vi "ReGenerate BFS Items.vi"(9 "Split Level":i32, 11 "Tree in":refnum<class "Tree.lvclass">) -> (0 "BFS Items Array":cluster{"Array of Single Level":T1[]}[](array[cluster]), 2 "Split Out":T1[](array[typedef]), 3 "Tree out":refnum<class "Tree.lvclass">)   [LabVIEW 2024, in "Tree.lvclass"]
uses:
  Tree.lvclass
  Type Def/Single Level.ctl
  Type Def/Tree Item.ctl
  Tree.lvclass/Tree.ctl
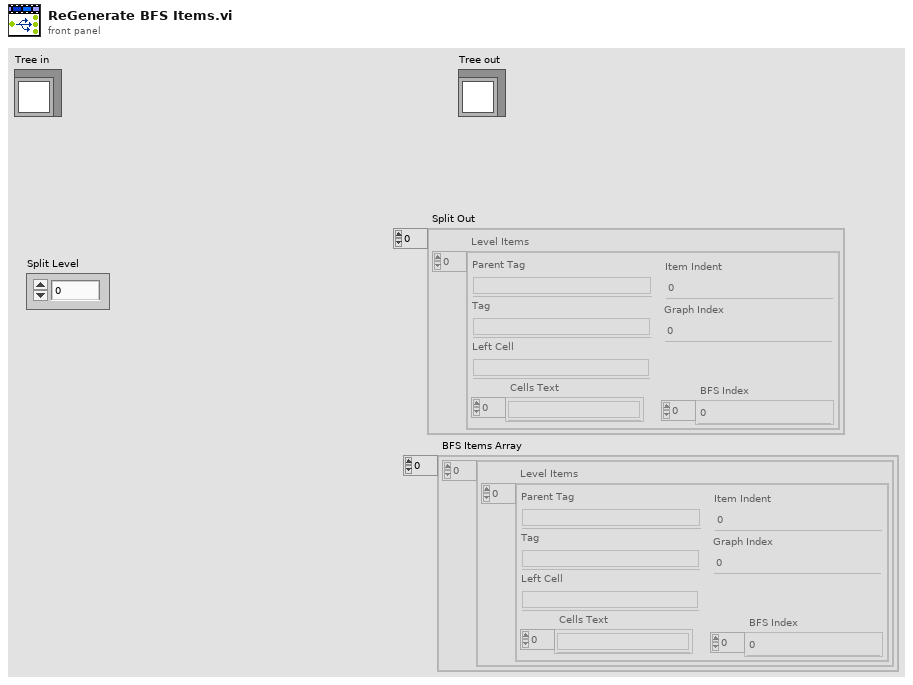
[diagram p1: front panel]
types:
  T1 = typedef "Single Level.ctl" = cluster{"Level Items":T2[]}
  T2 = typedef "Tree Item.ctl" = cluster{"Parent Tag":string, "Tag":string, "Left Cell":string, "Cells Text":string[], "BFS Index":i32[], "Graph Index":i32, "Item Indent":i32}
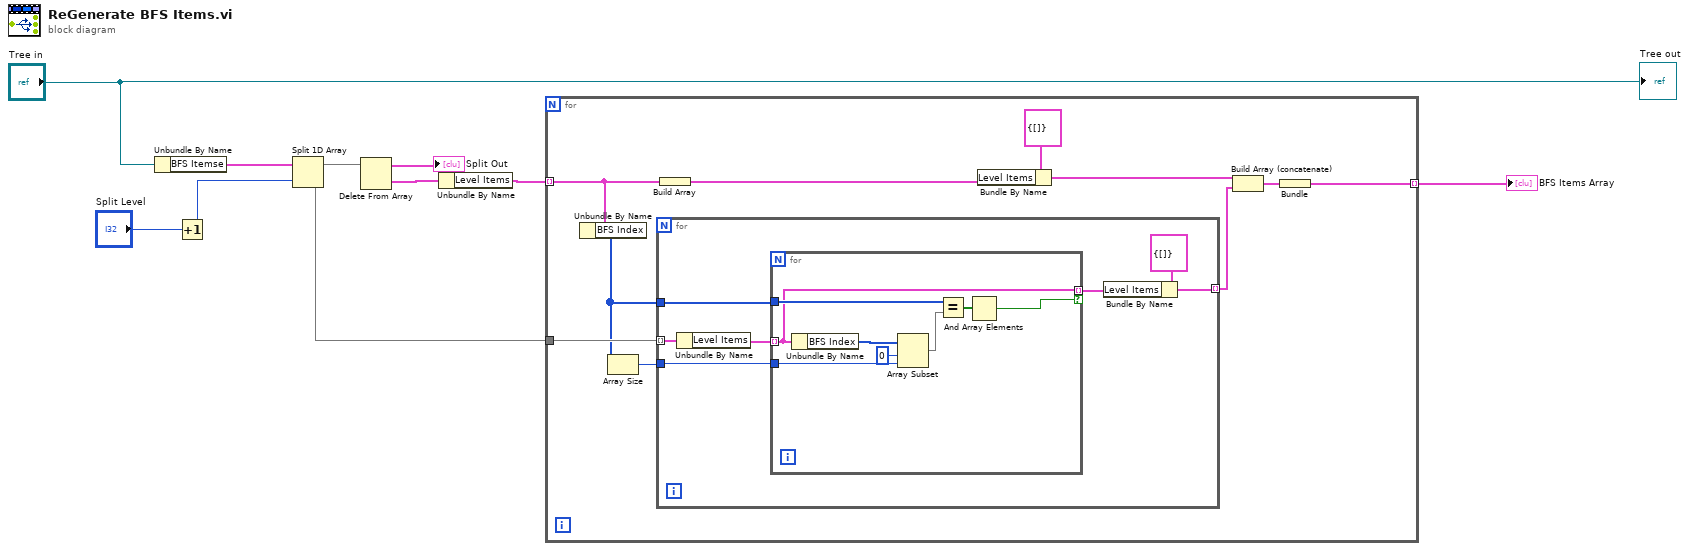
[diagram p0: block diagram]
diagram:
  n1 = Unbundle By Name("Tree in") -> ("BFS Itemse"=w8:T1[])
  n2 = Increment(x="Split Level") -> (x+1=w7:i32)
  n3 = Split 1D Array(array=w8, index=w7) -> (first subarray=w4:T1[], second subarray=w5:T1[])
  n4 = Delete From Array(array=w4) -> (deleted portion=w3:T1, array with subset deleted=→"Split Out":T1[])  [unwired: 2 in]
  n5 = Unbundle By Name(w3) -> ("Level Items"=w6:T2[])
  n6 = for {
    tunnel: w6 -> [w19] mode=indexing
    tunnel: w5 -> [w20]
    tunnel: [w14] -> w1 mode=indexing
    n7 = Unbundle By Name(w19) -> ("BFS Index"=w12:i32[])
    n8 = Array Size(array=w12) -> (size(s)=w13:i32)
    n9 = for {
      tunnel: w20 -> [w27] mode=indexing
      tunnel: w13 -> [w25]
      tunnel: w12 -> [w24]
      tunnel: [w21] -> w11 mode=indexing
      n10 = Unbundle By Name(w27) -> ("Level Items"=w26:T2[])
      n11 = for {
        tunnel: w26 -> [w29] mode=indexing
        tunnel: w25 -> [w33]
        tunnel: w24 -> [w31]
        tunnel: [w29] -> w23 mode=indexing if=w28
        n12 = Unbundle By Name(w29) -> ("BFS Index"=w35:i32[])
        n13 = Array Subset(array=w35, index=0, length=w33) -> (w32:i32[])
        n14 = Equal?(x=w31, y=w32) -> (x = y?=w30:bool[])
        n15 = And Array Elements(Boolean array=w30) -> (logical AND=w28:bool)
      }
      n16 = Bundle By Name(cluster=T1 {"Level Items"=[]} ("element"), "Level Items"=w23) -> (w21:T1)
    }
    n17 = Build Array(w19) -> (w18:T2[])
    n18 = Bundle By Name(cluster=T1 {"Level Items"=[]} ("element"), "Level Items"=w18) -> (w16:T1)
    n19 = Build Array (concatenate)(w16, w11) -> (w15:T1[])
    n20 = Bundle(w15) -> (w14:cluster{T1[]})  [unwired: 1 in]
  }
  "BFS Items Array" <- w1
  "Tree out" <- "Tree in"
